vi "GetPIDAngleGains.vi"(8 "error in (no error)":errorcluster) -> (0 "error out":errorcluster, 2 "Angle PID gains":T1)   [LabVIEW 2016, in "DriveBase.lvclass"]
uses:
  DriveBase.lvclass
  DriveBase.lvclass/DriveBase.ctl
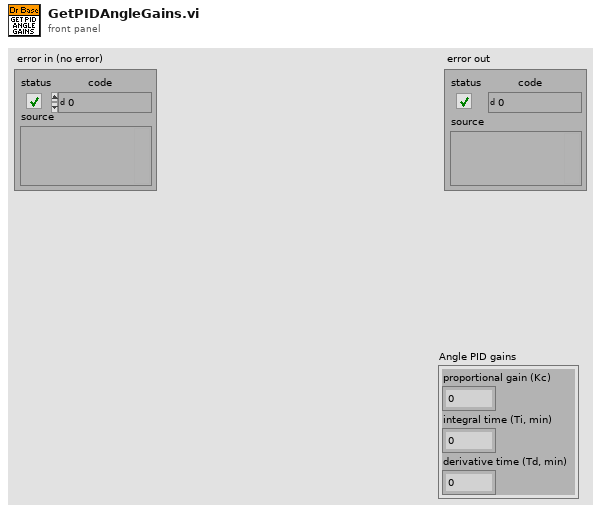
[diagram p1: front panel]
types:
  T1 = cluster{"proportional gain (Kc)":dbl, "integral time (Ti, min)":dbl, "derivative time (Td, min)":dbl}
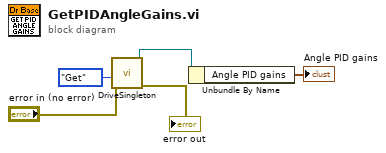
[diagram p0: block diagram]
diagram:
  n1 = call "DriveSingleton.vi"("error in (no error)"="error in (no error)", "Get/Set"=enum16{"Get", "Set"}."Get") -> ("error out"=→"error out":errorcluster, "DriveBase.lvclass 2"=w3:refnum<class "DriveBase.lvclass">)  [unwired: 8 in]
  n2 = Unbundle By Name(w3) -> ("Angle PID gains"=→"Angle PID gains":T1)
